vi "Read Child Name.vi"(8 "error in (no error)":errorcluster, 11 "[MDI] Child in":refnum<class "[MDI] Child.lvclass">) -> (0 "error out":errorcluster, 2 "child name":string, 3 "[MDI] Child out":refnum<class "[MDI] Child.lvclass">)   [LabVIEW 2020, in "[MDI] Child.lvlib" / "[MDI] Child.lvclass"]
uses:
  [MDI] Child.lvclass
  [MDI] Child.lvclass/[MDI] Child.ctl
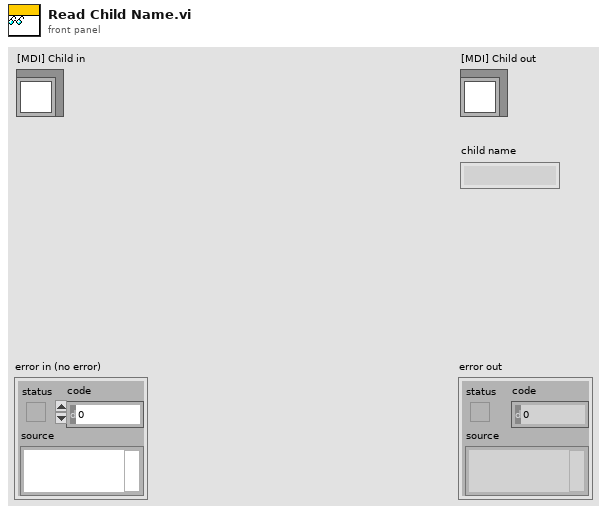
[diagram p1: front panel]
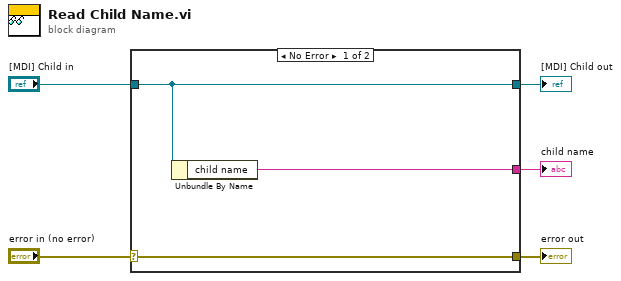
[diagram p0: block diagram]
diagram:
  n1 = case shown="No Error" "error in (no error)" {
    selector: "error in (no error)" -> [w8 w9]
    tunnel: [w8 w9] -> w4
    tunnel: [w7 w10] -> w2
    tunnel: "[MDI] Child in" -> [w7 w10]
    tunnel: [w6 _] -> w1
    frame No Error {
      n2 = Unbundle By Name(w7) -> ("child name"=w6:string)
    }
    frame Error {
    }
  }
  "error out" <- w4
  "[MDI] Child out" <- w2
  "child name" <- w1
